vi "Dash Read.vi"(2 "PID gains A":T1={"proportional gain (Kc)"=0.039, "integral time (Ti, min)"=0.0, "derivative time (Td, min)"=0.0018000000000000004} {"derivative time (Td, min)" format="%.4f"; "integral time (Ti, min)" format="%.4f"; "proportional gain (Kc)" format="%.4f"}, 3 "PID gains B":T1={"proportional gain (Kc)"=0.027999999999999997, "integral time (Ti, min)"=0.0, "derivative time (Td, min)"=0.0018000000000000004} {"derivative time (Td, min)" format="%.4f"; "integral time (Ti, min)" format="%.4f"; "proportional gain (Kc)" format="%.4f"}, 18 "Auto Options":T5={"Starting Position"=enum."Left L1 ", "First Score Pos"=enum."7", "Second Score Pos"=enum."5"}) -> (12 "Competion":string, 14 "Replay Number":dbl, 15 "Match Number":dbl, 16 "Match Type":string, 17 "output cluster":T2, 19 "AutoValid?":bool)   [LabVIEW 2018]
uses:
  Subsystems/Drive/MotionProfile/StartingPosition.ctl
  Subsystems/Drive/MotionProfile/Path_Decider.ctl
  <vilib>/Rock Robotics/Network Tables/NT Read Boolean.vi
  <vilib>/Rock Robotics/Network Tables/NT Write Variant.vi
  <vilib>/Rock Robotics/Network Tables/NT Read Number.vi
  <vilib>/Rock Robotics/Network Tables/NT Read Numeric Array.vi
  <vilib>/Rock Robotics/Network Tables/NT Read String.vi
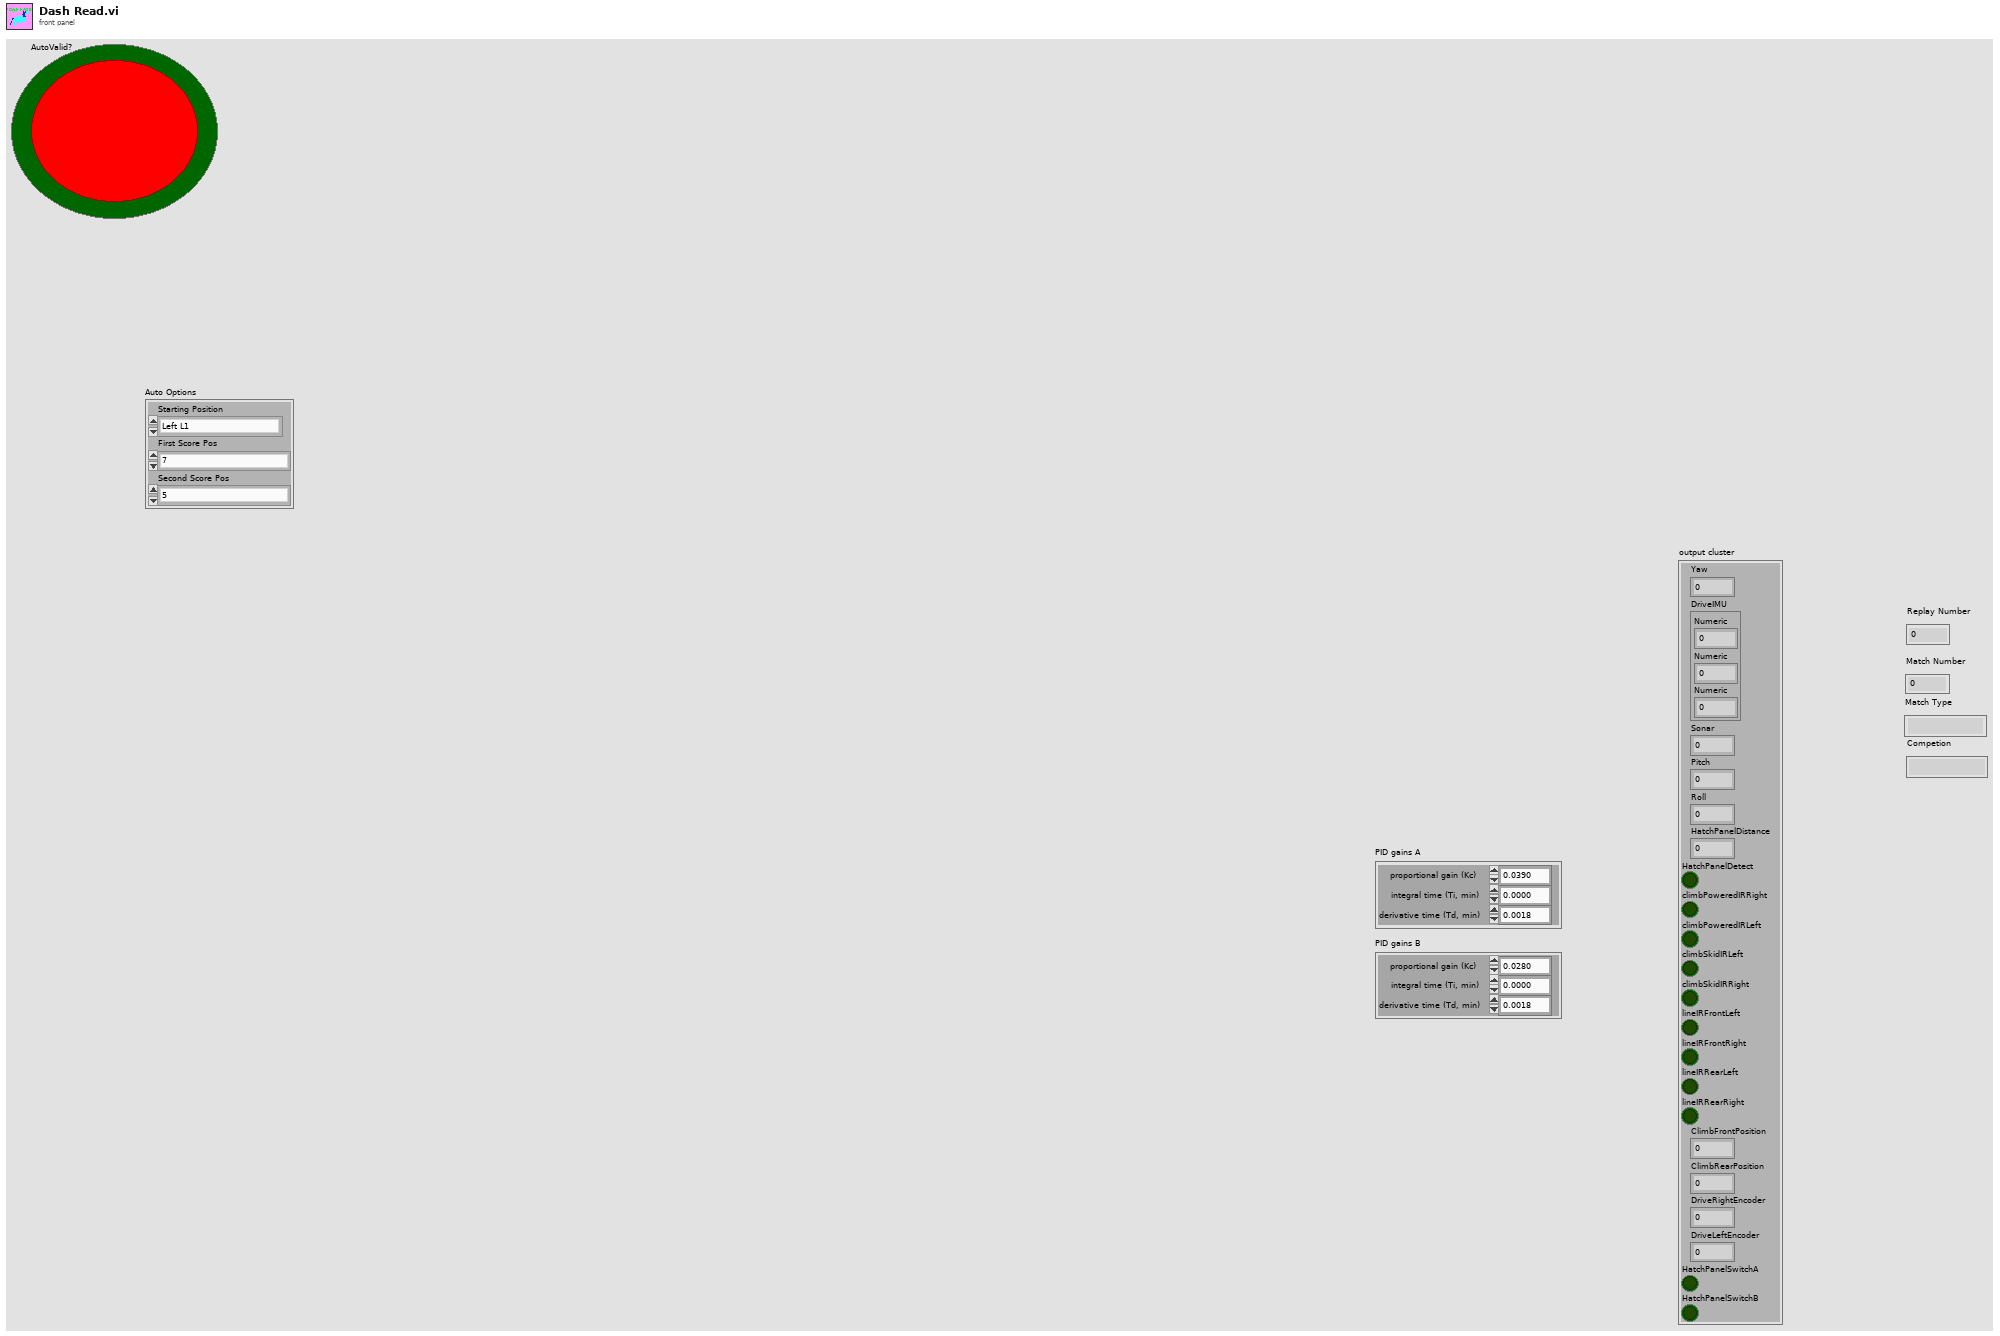
[diagram p1: front panel]
types:
  T1 = cluster{"proportional gain (Kc)":dbl, "integral time (Ti, min)":dbl, "derivative time (Td, min)":dbl}
  T2 = cluster{"Yaw":dbl, "DriveIMU":cluster{"Numeric":dbl, "Numeric":dbl, "Numeric":dbl}, "Sonar":dbl, "Pitch":dbl, "Roll":dbl, "HatchPanelDistance":dbl, "HatchPanelDetect":bool, "climbPoweredIRRight":bool, "climbPoweredIRLeft":bool, "climbSkidIRLeft":bool, "climbSkidIRRight":bool, "lineIRFrontLeft":bool, "lineIRFrontRight":bool, "lineIRRearLeft":bool, "lineIRRearRight":bool, "ClimbFrontPosition":dbl, "ClimbRearPosition":dbl, "DriveRightEncoder":dbl, "DriveLeftEncoder":dbl, "HatchPanelSwitchA":bool, "HatchPanelSwitchB":bool}
  T3 = typedef "StartingPosition.ctl" = enum16{"Left L1 ", "Middle L1", "Right L1", "Left L2", "Right L2", "Don't Move"}
  T4 = typedef "Path_Decider.ctl" = enum16{"1", "2", "3", "4", "5", "6", "7", "8", "Left_Rocket_Front", "Left_Rocket_Rear", "Right_Rocket_Front", "Right_Rocket_Rear"}
  T5 = cluster{"Starting Position":T3, "First Score Pos":T4, "Second Score Pos":T4}
  T6 = cluster{"Numeric":dbl, "Numeric":dbl, "Numeric":dbl}
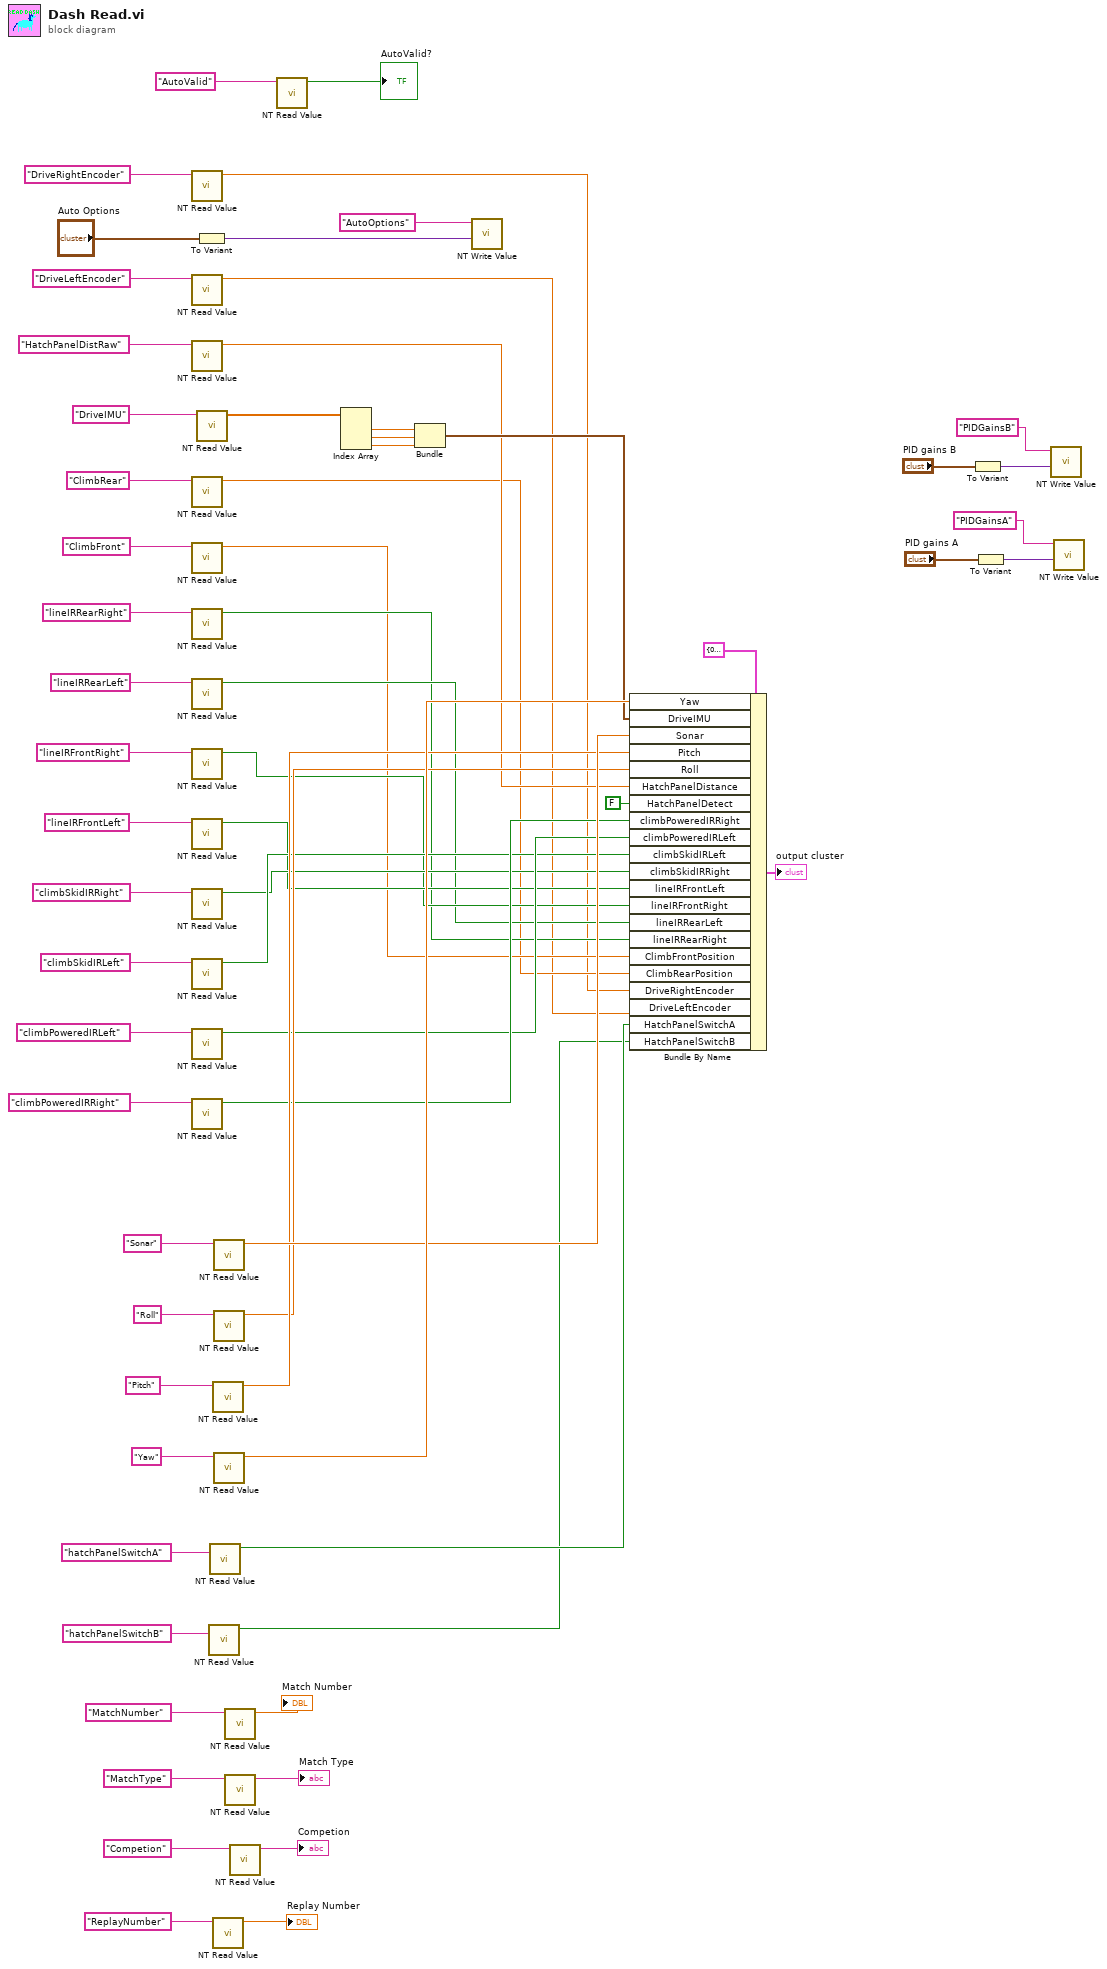
[diagram p0: block diagram]
diagram:
  n1 = call-poly <vilib>:"NT Read Value.vi"("Name"="DriveRightEncoder") -> ("Numeric"=w23:dbl)  [unwired: 9 in, 1 out]
  n2 = call-poly <vilib>:"NT Read Value.vi"("Name"="DriveLeftEncoder") -> ("Numeric"=w22:dbl)  [unwired: 9 in, 1 out]
  n3 = call-poly <vilib>:"NT Read Value.vi"("Name"="HatchPanelDistRaw") -> ("Numeric"=w34:dbl)  [unwired: 9 in, 1 out]
  n4 = call-poly <vilib>:"NT Read Value.vi"("Name"="ClimbRear") -> ("Numeric"=w24:dbl)  [unwired: 9 in, 1 out]
  n5 = call-poly <vilib>:"NT Read Value.vi"("Name"="ClimbFront") -> ("Numeric"=w25:dbl)  [unwired: 9 in, 1 out]
  n6 = call-poly <vilib>:"NT Read Value.vi"("Name"="lineIRRearRight") -> ("Boolean"=w26:bool)  [unwired: 9 in, 1 out]
  n7 = call-poly <vilib>:"NT Read Value.vi"("Name"="lineIRRearLeft") -> ("Boolean"=w27:bool)  [unwired: 9 in, 1 out]
  n8 = call-poly <vilib>:"NT Read Value.vi"("Name"="lineIRFrontRight") -> ("Boolean"=w28:bool)  [unwired: 9 in, 1 out]
  n9 = call-poly <vilib>:"NT Read Value.vi"("Name"="lineIRFrontLeft") -> ("Boolean"=w29:bool)  [unwired: 9 in, 1 out]
  n10 = call-poly <vilib>:"NT Read Value.vi"("Name"="climbSkidIRRight") -> ("Boolean"=w30:bool)  [unwired: 9 in, 1 out]
  n11 = call-poly <vilib>:"NT Read Value.vi"("Name"="climbSkidIRLeft") -> ("Boolean"=w31:bool)  [unwired: 9 in, 1 out]
  n12 = call-poly <vilib>:"NT Read Value.vi"("Name"="climbPoweredIRLeft") -> ("Boolean"=w32:bool)  [unwired: 9 in, 1 out]
  n13 = call-poly <vilib>:"NT Read Value.vi"("Name"="climbPoweredIRRight") -> ("Boolean"=w33:bool)  [unwired: 9 in, 1 out]
  n14 = To Variant(anything="Auto Options") -> (Variant=w56:variant)
  n15 = call-poly <vilib>:"NT Read Value.vi"("Name"="DriveIMU") -> ("Numeric Array"=w43:dbl[])  [unwired: 9 in, 1 out]
  n16 = call-poly <vilib>:"NT Read Value.vi"("Name"="hatchPanelSwitchB") -> ("Boolean"=w18:bool)  [unwired: 9 in, 1 out]
  n17 = call-poly <vilib>:"NT Read Value.vi"("Name"="hatchPanelSwitchA") -> ("Boolean"=w19:bool)  [unwired: 9 in, 1 out]
  n18 = call-poly <vilib>:"NT Read Value.vi"("Name"="Pitch") -> ("Numeric"=w36:dbl)  [unwired: 9 in, 1 out]
  n19 = call-poly <vilib>:"NT Read Value.vi"("Name"="ReplayNumber") -> ("Numeric"=→"Replay Number":dbl)  [unwired: 9 in, 1 out]
  n20 = call-poly <vilib>:"NT Read Value.vi"("Name"="Sonar") -> ("Numeric"=w37:dbl)  [unwired: 9 in, 1 out]
  n21 = call-poly <vilib>:"NT Read Value.vi"("Name"="Roll") -> ("Numeric"=w35:dbl)  [unwired: 9 in, 1 out]
  n22 = call-poly <vilib>:"NT Read Value.vi"("Name"="Yaw") -> ("Numeric"=w39:dbl)  [unwired: 9 in, 1 out]
  n23 = call-poly <vilib>:"NT Read Value.vi"("Name"="MatchNumber") -> ("Numeric"=→"Match Number":dbl)  [unwired: 9 in, 1 out]
  n24 = call-poly <vilib>:"NT Read Value.vi"("Name"="MatchType") -> ("String"=→"Match Type":string)  [unwired: 9 in, 1 out]
  n25 = call-poly <vilib>:"NT Read Value.vi"("Name"="Competion") -> ("String"=→"Competion":string)  [unwired: 9 in, 1 out]
  n26 = call-poly <vilib>:"NT Read Value.vi"("Name"="AutoValid") -> ("Boolean"=→"AutoValid?":bool)  [unwired: 9 in, 1 out]
  n27 = Index Array(array=w43) -> (element #1=w42:dbl, element #2=w41:dbl, element #3=w40:dbl)  [unwired: 3 in]
  n28 = Bundle("Numeric"=w42, "Numeric"=w41, "Numeric"=w40) -> (w38:T6)  [unwired: 1 in]
  n29 = call-poly <vilib>:"NT Write Value.vi"("Variant"=w56, "Name"="AutoOptions") -> ()  [unwired: 9 in, 1 out]
  n30 = Bundle By Name(cluster=T2 {"Yaw"=0.0, "DriveIMU"={"Numeric"=0.0, "Numeric"=0.0, "Numeric"=0.0}, "Sonar"=0.0, "Pitch"=0.0, "Roll"=0.0, "HatchPanelDistance"=0.0, "HatchPanelDetect"=FALSE, "climbPoweredIRRight"=FALSE, "climbPoweredIRLeft"=FALSE, "climbSkidIRLeft"=FALSE, "climbSkidIRRight"=FALSE, "lineIRFrontLeft"=FALSE, "lineIRFrontRight"=FALSE, "lineIRRearLeft"=FALSE, "lineIRRearRight"=FALSE, "ClimbFrontPosition"=0.0, "ClimbRearPosition"=0.0, "DriveRightEncoder"=0.0, "DriveLeftEncoder"=0.0, "HatchPanelSwitchA"=FALSE, "HatchPanelSwitchB"=FALSE} ("Important Robot Data"), "Yaw"=w39, "DriveIMU"=w38, "Sonar"=w37, "Pitch"=w36, "Roll"=w35, "HatchPanelDistance"=w34, "HatchPanelDetect"=FALSE, "climbPoweredIRRight"=w33, "climbPoweredIRLeft"=w32, "climbSkidIRLeft"=w31, "climbSkidIRRight"=w30, "lineIRFrontLeft"=w29, "lineIRFrontRight"=w28, "lineIRRearLeft"=w27, "lineIRRearRight"=w26, "ClimbFrontPosition"=w25, "ClimbRearPosition"=w24, "DriveRightEncoder"=w23, "DriveLeftEncoder"=w22, "HatchPanelSwitchA"=w19, "HatchPanelSwitchB"=w18) -> (→"output cluster":T2)
  n31 = To Variant(anything="PID gains B") -> (Variant=w11:variant)
  n32 = To Variant(anything="PID gains A") -> (Variant=w13:variant)
  n33 = call-poly <vilib>:"NT Write Value.vi"("Variant"=w11, "Name"="PIDGainsB") -> ()  [unwired: 9 in, 1 out]
  n34 = call-poly <vilib>:"NT Write Value.vi"("Variant"=w13, "Name"="PIDGainsA") -> ()  [unwired: 9 in, 1 out]
